vi "MDAQ_SurfaceHistogram.vi"(10 "Surface In":dbl[][](array[numeric]), 11 "Surface CV PlotRef":refnum<vi>) -> (2 "Surface Out":dbl[][](array[numeric]))   [LabVIEW 2021]
uses:
  <vilib>/Analysis/NI_AALBase.lvlib
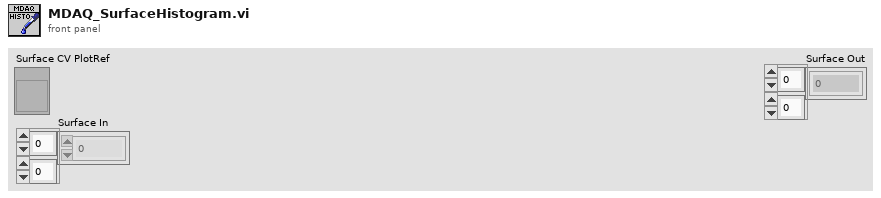
[diagram p1: front panel]
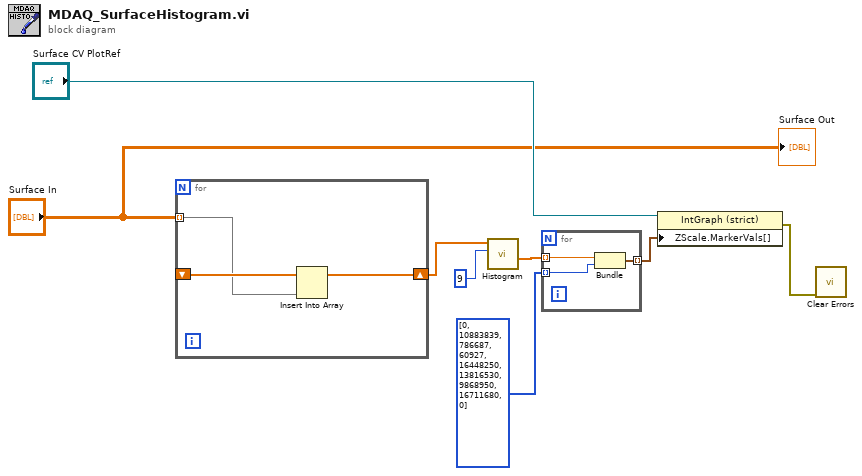
[diagram p0: block diagram]
diagram:
  n1 = for {
    tunnel: "Surface In" -> [w9] mode=indexing
    shift-right: [w10] -> w7
    shift-left: _ -> [w11]
    n2 = Insert Into Array(array=w11, new element=w9) -> (w10:dbl[])  [unwired: 1 in]
  }
  n3 = call <vilib>:"Histogram.vi"("intervals"=9, "X"=w7) -> ("X Values"=w5:dbl[])  [unwired: 6 in, 3 out]
  n4 = for {
    tunnel: [w14] -> w3 mode=indexing
    tunnel: w5 -> [w13] mode=indexing
    tunnel: u32[] [0, 10883839, 786687, 60927, 16448250, 13816530, 9868950, 16711680, 0] -> [w12] mode=indexing
    n5 = Bundle(w13, w12) -> (w14:cluster{dbl, u32})  [unwired: 1 in]
  }
  n6 = property class="IntGraph (strict)"(reference="Surface CV PlotRef", "ZScale.MarkerVals[]"=w3) -> (error out=w1:errorcluster)  [unwired: 1 in, 1 out]
  n7 = call <vilib>:"Clear Errors.vi"("error in (no error)"=w1) -> ()  [unwired: 5 in, 2 out]
  "Surface Out" <- "Surface In"
